vi "Select or Save Path Configuration.vi"(7 "Action (0: Select)":i32(ring) items=["Select", "Save"], 8 "error in (no error)":errorcluster, 9 "Configuration Name (\"Default\")":string="Default", 10 "Channel (1)":i32=1, 11 "VISA resource name":refnum<visa-resource-name>) -> (0 "error out":errorcluster, 3 "VISA resource name out":refnum<visa-resource-name>)   [LabVIEW 2018, in "Keysight PNA Series.lvlib"]
doc: "Loads the named configuration onto the specified channel, or saves the path configuration currently associated with the specified channel to the specified configuration name."
uses:
  Keysight PNA Series.lvlib
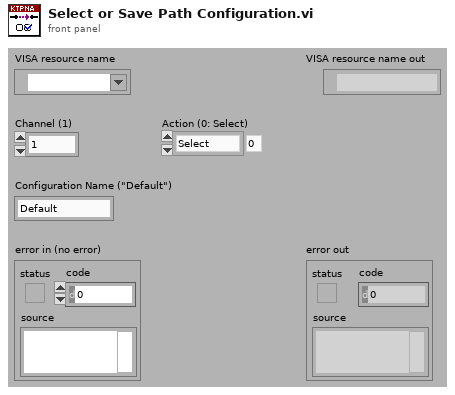
[diagram p1: front panel]
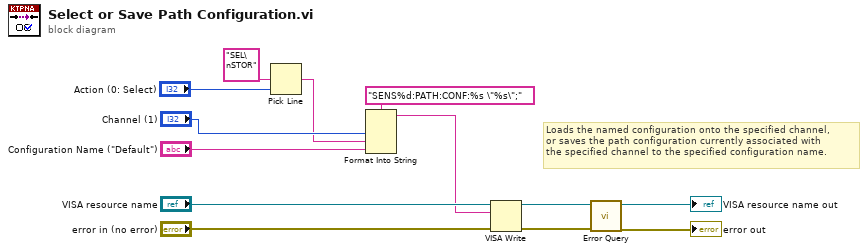
[diagram p0: block diagram]
diagram:
  # "Loads the named configuration onto the specified channel,\nor saves the path configuration currently associated with\nthe specified channel to the specified configuration name."
  n1 = Pick Line(multi-line string="SEL\nSTOR", line index="Action (0: Select)") -> (output string=w2:string)  [unwired: 1 in]
  n2 = Format Into String(format string="SENS%d:PATH:CONF:%s \"%s\";", "Channel (1)", w2, "Configuration Name (\"Default\")") -> (resulting string=w1:string)  [unwired: 2 in, 1 out]
  n3 = VISA Write(VISA resource name="VISA resource name", write buffer=w1, error in (no error)="error in (no error)") -> (VISA resource name out=w9:refnum<visa-resource-name>, error out=w8:errorcluster)  [unwired: 1 out]
  n4 = call "Error Query.vi"("error in (no error)"=w8, "VISA resource name"=w9) -> ("error out"=→"error out":errorcluster, "VISA resource name out"=→"VISA resource name out":refnum<visa-resource-name>)  [unwired: 6 in, 2 out]
